vi "solar_addon QTimers Add.vi"(8 "error in (no error)":errorcluster) -> (0 "error out":errorcluster, 1 "Cancelled":bool, 2 "Target out":string, 3 "QTimer out":string)   [LabVIEW 2018]
doc: "This dialog adds a new QTimer interface."
uses:
  <vilib>/Utility/miscctls.llb/LVSelectionTypeDef.ctl
panel:
  in  "Cancel":bool
  in  "OK":bool
  in  "Target":string
  in  "QTimer":string
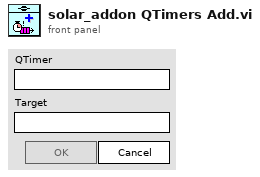
[diagram p1: front panel]
types:
  T1 = typedef "LVSelectionTypeDef.ctl" = cluster{"Selection Start":u32, "Selection End":u32}
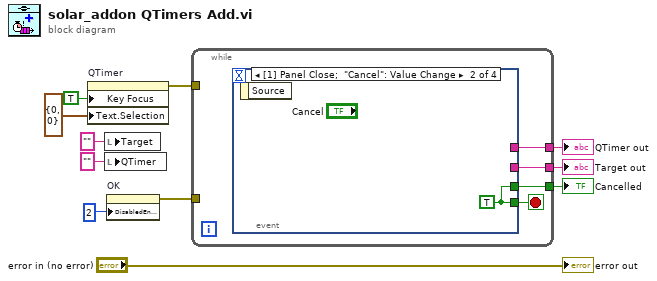
[diagram p0: block diagram]
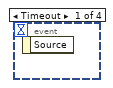
[diagram p2: hidden frame]
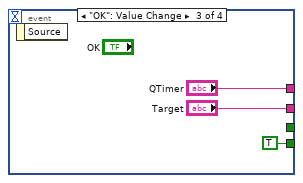
[diagram p3: hidden frame]
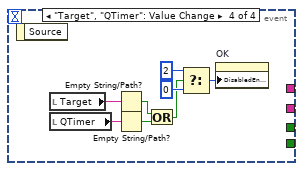
[diagram p4: hidden frame]
diagram:
  n1 = property on="QTimer" class="Str"("Key Focus"=TRUE, "Text.Selection"=T1 {"Selection Start"=0, "Selection End"=0}) -> (error out=w1:errorcluster)  [unwired: 2 in, 1 out]
  n2 = local write "Target"("" ("Target")) -> ()
  n3 = local write "QTimer"("" ("QTimer")) -> ()
  n4 = property on="OK" class="Bool"("DisabledEnum"=u8 2) -> (error out=w5:errorcluster)  [unwired: 2 in, 1 out]
  n5 = while {
    tunnel: [w14] -> w10
    tunnel: [w13] -> w7
    tunnel: w5 -> [_]
    tunnel: [w12] -> w4
    tunnel: w1 -> [_]
    stop <- w15 stop-if-true
    n6 = event shown="[1] Panel Close;  \"Cancel\": Value Change" {
      selector: _ -> [_ _ _ _]
      dyn-events: _ -> [_ _ _ _]
      timeout: _ -> [_ _ _ _]
      tunnel: [_ w16 TRUE _] -> w15
      tunnel: [_ w16 _ _] -> w14
      tunnel: [_ _ "QTimer" _] -> w13
      tunnel: [_ _ "Target" _] -> w12
      event Timeout {
        n7 = event-data() -> ()  [unwired: 1 in, 1 out]
      }
      event Panel Close; "Cancel": Value Change {
        w16 = TRUE
        n8 = event-data() -> ()  [unwired: 1 in, 1 out]
      }
      event "OK": Value Change {
        n9 = event-data() -> ()  [unwired: 1 in, 1 out]
      }
      event "Target", "QTimer": Value Change {
        n10 = event-data() -> ()  [unwired: 1 in, 1 out]
        n11 = local read "Target"() -> (w27:string)
        n12 = local read "QTimer"() -> (w26:string)
        n13 = Empty String/Path?(string/path=w27) -> (empty?=w24:bool)
        n14 = Empty String/Path?(string/path=w26) -> (empty?=w25:bool)
        n15 = Or(x=w24, y=w25) -> (x .or. y?=w20:bool)
        n16 = Select(t=u8 2, s=w20, f=u8 0) -> (s? t:f=w21:u8)
        n17 = property on="OK" class="Bool"("DisabledEnum"=w21) -> ()  [unwired: 2 in, 2 out]
      }
    }
  }
  "Cancelled" <- w10
  "QTimer out" <- w7
  "Target out" <- w4
  "error out" <- "error in (no error)"
